vi "etc_XCITE_GetXCStruct.vi"(8 "error in (no error)":errorcluster {"code" format="%x"}, 11 "h":u64) -> (0 "error out":errorcluster {"code" format="%x"}, 1 "XCiteStructure":T1, 2 "ErrorMessage":i32 format="%x", 3 "h out":u64)   [LabVIEW 2019, in "XCite.lvlib"]
doc: "Gets the Xcite structure from the device with various properties."
uses:
  XCite.lvlib
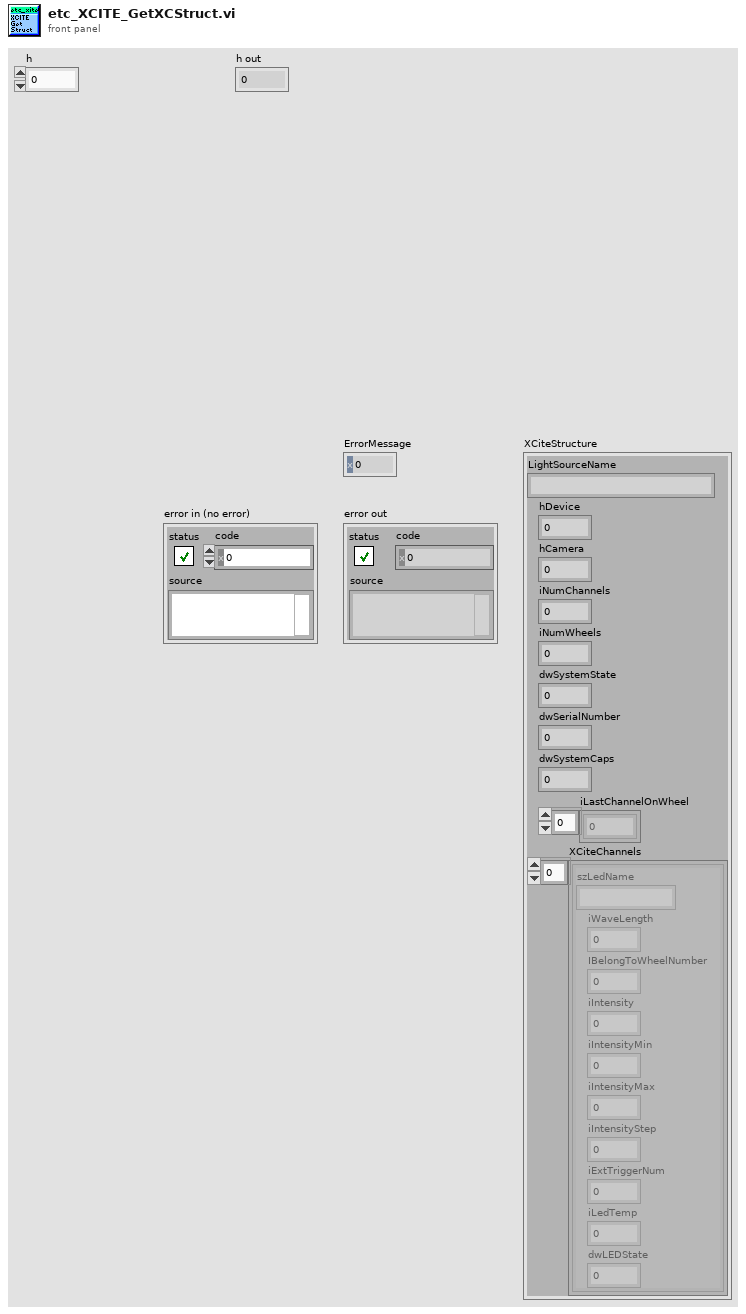
[diagram p1: front panel]
types:
  T1 = cluster{"LightSourceName":string, "hDevice":u64, "hCamera":u64, "iNumChannels":i32, "iNumWheels":i32, "dwSystemState":u32, "dwSerialNumber":u32, "dwSystemCaps":u32, "iLastChannelOnWheel":i16[], "XCiteChannels":cluster{"szLedName":string, "iWaveLength":i32, "IBelongToWheelNumber":i32, "iIntensity":i32, "iIntensityMin":i32, "iIntensityMax":i32, "iIntensityStep":i32, "iExtTriggerNum":i32, "iLedTemp":i32, "dwLEDState":u32}[]}
  T2 = cluster{"wSize":u16, "czLightSourceName":cluster{u8, u8, u8, u8, u8, u8, u8, u8, u8, u8, u8, u8, u8, u8, u8, u8, u8, u8, u8, u8, u8, u8, u8, u8, u8, u8, u8, u8, u8, u8}, "hDevice":u64, "hCamera":u64, "iNumChannels":i32, "iNumWheels":i32, "dwSystemState":u32, "dwSerialNumber":u32, "dwSystemCaps":u32, "iLastChannelOnWheel":cluster{i32, i32, i32, i32, i32}, "ZZdwDummy":cluster{u32, u32, u32, u32, u32, u32, u32, u32, u32, u32, u32, u32, u32, u32, u32, u32}, "XCiteChannels":cluster{"XCiteC_raw":cluster{"szLedName":cluster{u8, u8, u8, u8, u8, u8, u8, u8, u8, u8, u8, u8, u8, u8, u8, u8}, "iWaveLength":i32, "IBelongToWheelNumber":i32, "iIntensity":i32, "iIntensityMin":i32, "iIntensityMax":i32, "iIntensityStep":i32, "iExtTriggerNum":i32, "iLedTemp":i32, "dwLEDState":u32, "ZZdwdummy":cluster{u32, u32, u32, u32, u32, u32, u32, u32, u32, u32, u32, u32, u32, u32, u32, u32}}, "XCiteC_raw":cluster{"szLedName":cluster{u8, u8, u8, u8, u8, u8, u8, u8, u8, u8, u8, u8, u8, u8, u8, u8}, "iWaveLength":i32, "IBelongToWheelNumber":i32, "iIntensity":i32, "iIntensityMin":i32, "iIntensityMax":i32, "iIntensityStep":i32, "iExtTriggerNum":i32, "iLedTemp":i32, "dwLEDState":u32, "ZZdwdummy":cluster{u32, u32, u32, u32, u32, u32, u32, u32, u32, u32, u32, u32, u32, u32, u32, u32}}, "XCiteC_raw":cluster{"szLedName":cluster{u8, u8, u8, u8, u8, u8, u8, u8, u8, u8, u8, u8, u8, u8, u8, u8}, "iWaveLength":i32, "IBelongToWheelNumber":i32, "iIntensity":i32, "iIntensityMin":i32, "iIntensityMax":i32, "iIntensityStep":i32, "iExtTriggerNum":i32, "iLedTemp":i32, "dwLEDState":u32, "ZZdwdummy":cluster{u32, u32, u32, u32, u32, u32, u32, u32, u32, u32, u32, u32, u32, u32, u32, u32}}, "XCiteC_raw":cluster{"szLedName":cluster{u8, u8, u8, u8, u8, u8, u8, u8, u8, u8, u8, u8, u8, u8, u8, u8}, "iWaveLength":i32, "IBelongToWheelNumber":i32, "iIntensity":i32, "iIntensityMin":i32, "iIntensityMax":i32, "iIntensityStep":i32, "iExtTriggerNum":i32, "iLedTemp":i32, "dwLEDState":u32, "ZZdwdummy":cluster{u32, u32, u32, u32, u32, u32, u32, u32, u32, u32, u32, u32, u32, u32, u32, u32}}, "XCiteC_raw":cluster{"szLedName":cluster{u8, u8, u8, u8, u8, u8, u8, u8, u8, u8, u8, u8, u8, u8, u8, u8}, "iWaveLength":i32, "IBelongToWheelNumber":i32, "iIntensity":i32, "iIntensityMin":i32, "iIntensityMax":i32, "iIntensityStep":i32, "iExtTriggerNum":i32, "iLedTemp":i32, "dwLEDState":u32, "ZZdwdummy":cluster{u32, u32, u32, u32, u32, u32, u32, u32, u32, u32, u32, u32, u32, u32, u32, u32}}, "XCiteC_raw":cluster{"szLedName":cluster{u8, u8, u8, u8, u8, u8, u8, u8, u8, u8, u8, u8, u8, u8, u8, u8}, "iWaveLength":i32, "IBelongToWheelNumber":i32, "iIntensity":i32, "iIntensityMin":i32, "iIntensityMax":i32, "iIntensityStep":i32, "iExtTriggerNum":i32, "iLedTemp":i32, "dwLEDState":u32, "ZZdwdummy":cluster{u32, u32, u32, u32, u32, u32, u32, u32, u32, u32, u32, u32, u32, u32, u32, u32}}, "XCiteC_raw":cluster{"szLedName":cluster{u8, u8, u8, u8, u8, u8, u8, u8, u8, u8, u8, u8, u8, u8, u8, u8}, "iWaveLength":i32, "IBelongToWheelNumber":i32, "iIntensity":i32, "iIntensityMin":i32, "iIntensityMax":i32, "iIntensityStep":i32, "iExtTriggerNum":i32, "iLedTemp":i32, "dwLEDState":u32, "ZZdwdummy":cluster{u32, u32, u32, u32, u32, u32, u32, u32, u32, u32, u32, u32, u32, u32, u32, u32}}, "XCiteC_raw":cluster{"szLedName":cluster{u8, u8, u8, u8, u8, u8, u8, u8, u8, u8, u8, u8, u8, u8, u8, u8}, "iWaveLength":i32, "IBelongToWheelNumber":i32, "iIntensity":i32, "iIntensityMin":i32, "iIntensityMax":i32, "iIntensityStep":i32, "iExtTriggerNum":i32, "iLedTemp":i32, "dwLEDState":u32, "ZZdwdummy":cluster{u32, u32, u32, u32, u32, u32, u32, u32, u32, u32, u32, u32, u32, u32, u32, u32}}, "XCiteC_raw":cluster{"szLedName":cluster{u8, u8, u8, u8, u8, u8, u8, u8, u8, u8, u8, u8, u8, u8, u8, u8}, "iWaveLength":i32, "IBelongToWheelNumber":i32, "iIntensity":i32, "iIntensityMin":i32, "iIntensityMax":i32, "iIntensityStep":i32, "iExtTriggerNum":i32, "iLedTemp":i32, "dwLEDState":u32, "ZZdwdummy":cluster{u32, u32, u32, u32, u32, u32, u32, u32, u32, u32, u32, u32, u32, u32, u32, u32}}, "XCiteC_raw":cluster{"szLedName":cluster{u8, u8, u8, u8, u8, u8, u8, u8, u8, u8, u8, u8, u8, u8, u8, u8}, "iWaveLength":i32, "IBelongToWheelNumber":i32, "iIntensity":i32, "iIntensityMin":i32, "iIntensityMax":i32, "iIntensityStep":i32, "iExtTriggerNum":i32, "iLedTemp":i32, "dwLEDState":u32, "ZZdwdummy":cluster{u32, u32, u32, u32, u32, u32, u32, u32, u32, u32, u32, u32, u32, u32, u32, u32}}, "XCiteC_raw":cluster{"szLedName":cluster{u8, u8, u8, u8, u8, u8, u8, u8, u8, u8, u8, u8, u8, u8, u8, u8}, "iWaveLength":i32, "IBelongToWheelNumber":i32, "iIntensity":i32, "iIntensityMin":i32, "iIntensityMax":i32, "iIntensityStep":i32, "iExtTriggerNum":i32, "iLedTemp":i32, "dwLEDState":u32, "ZZdwdummy":cluster{u32, u32, u32, u32, u32, u32, u32, u32, u32, u32, u32, u32, u32, u32, u32, u32}}, "XCiteC_raw":cluster{"szLedName":cluster{u8, u8, u8, u8, u8, u8, u8, u8, u8, u8, u8, u8, u8, u8, u8, u8}, "iWaveLength":i32, "IBelongToWheelNumber":i32, "iIntensity":i32, "iIntensityMin":i32, "iIntensityMax":i32, "iIntensityStep":i32, "iExtTriggerNum":i32, "iLedTemp":i32, "dwLEDState":u32, "ZZdwdummy":cluster{u32, u32, u32, u32, u32, u32, u32, u32, u32, u32, u32, u32, u32, u32, u32, u32}}, "XCiteC_raw":cluster{"szLedName":cluster{u8, u8, u8, u8, u8, u8, u8, u8, u8, u8, u8, u8, u8, u8, u8, u8}, "iWaveLength":i32, "IBelongToWheelNumber":i32, "iIntensity":i32, "iIntensityMin":i32, "iIntensityMax":i32, "iIntensityStep":i32, "iExtTriggerNum":i32, "iLedTemp":i32, "dwLEDState":u32, "ZZdwdummy":cluster{u32, u32, u32, u32, u32, u32, u32, u32, u32, u32, u32, u32, u32, u32, u32, u32}}, "XCiteC_raw":cluster{"szLedName":cluster{u8, u8, u8, u8, u8, u8, u8, u8, u8, u8, u8, u8, u8, u8, u8, u8}, "iWaveLength":i32, "IBelongToWheelNumber":i32, "iIntensity":i32, "iIntensityMin":i32, "iIntensityMax":i32, "iIntensityStep":i32, "iExtTriggerNum":i32, "iLedTemp":i32, "dwLEDState":u32, "ZZdwdummy":cluster{u32, u32, u32, u32, u32, u32, u32, u32, u32, u32, u32, u32, u32, u32, u32, u32}}, "XCiteC_raw":cluster{"szLedName":cluster{u8, u8, u8, u8, u8, u8, u8, u8, u8, u8, u8, u8, u8, u8, u8, u8}, "iWaveLength":i32, "IBelongToWheelNumber":i32, "iIntensity":i32, "iIntensityMin":i32, "iIntensityMax":i32, "iIntensityStep":i32, "iExtTriggerNum":i32, "iLedTemp":i32, "dwLEDState":u32, "ZZdwdummy":cluster{u32, u32, u32, u32, u32, u32, u32, u32, u32, u32, u32, u32, u32, u32, u32, u32}}, "XCiteC_raw":cluster{"szLedName":cluster{u8, u8, u8, u8, u8, u8, u8, u8, u8, u8, u8, u8, u8, u8, u8, u8}, "iWaveLength":i32, "IBelongToWheelNumber":i32, "iIntensity":i32, "iIntensityMin":i32, "iIntensityMax":i32, "iIntensityStep":i32, "iExtTriggerNum":i32, "iLedTemp":i32, "dwLEDState":u32, "ZZdwdummy":cluster{u32, u32, u32, u32, u32, u32, u32, u32, u32, u32, u32, u32, u32, u32, u32, u32}}}}
  T3 = cluster{u8, u8, u8, u8, u8, u8, u8, u8, u8, u8, u8, u8, u8, u8, u8, u8, u8, u8, u8, u8, u8, u8, u8, u8, u8, u8, u8, u8, u8, u8}
  T4 = cluster{"XCiteC_raw":cluster{"szLedName":cluster{u8, u8, u8, u8, u8, u8, u8, u8, u8, u8, u8, u8, u8, u8, u8, u8}, "iWaveLength":i32, "IBelongToWheelNumber":i32, "iIntensity":i32, "iIntensityMin":i32, "iIntensityMax":i32, "iIntensityStep":i32, "iExtTriggerNum":i32, "iLedTemp":i32, "dwLEDState":u32, "ZZdwdummy":cluster{u32, u32, u32, u32, u32, u32, u32, u32, u32, u32, u32, u32, u32, u32, u32, u32}}, "XCiteC_raw":cluster{"szLedName":cluster{u8, u8, u8, u8, u8, u8, u8, u8, u8, u8, u8, u8, u8, u8, u8, u8}, "iWaveLength":i32, "IBelongToWheelNumber":i32, "iIntensity":i32, "iIntensityMin":i32, "iIntensityMax":i32, "iIntensityStep":i32, "iExtTriggerNum":i32, "iLedTemp":i32, "dwLEDState":u32, "ZZdwdummy":cluster{u32, u32, u32, u32, u32, u32, u32, u32, u32, u32, u32, u32, u32, u32, u32, u32}}, "XCiteC_raw":cluster{"szLedName":cluster{u8, u8, u8, u8, u8, u8, u8, u8, u8, u8, u8, u8, u8, u8, u8, u8}, "iWaveLength":i32, "IBelongToWheelNumber":i32, "iIntensity":i32, "iIntensityMin":i32, "iIntensityMax":i32, "iIntensityStep":i32, "iExtTriggerNum":i32, "iLedTemp":i32, "dwLEDState":u32, "ZZdwdummy":cluster{u32, u32, u32, u32, u32, u32, u32, u32, u32, u32, u32, u32, u32, u32, u32, u32}}, "XCiteC_raw":cluster{"szLedName":cluster{u8, u8, u8, u8, u8, u8, u8, u8, u8, u8, u8, u8, u8, u8, u8, u8}, "iWaveLength":i32, "IBelongToWheelNumber":i32, "iIntensity":i32, "iIntensityMin":i32, "iIntensityMax":i32, "iIntensityStep":i32, "iExtTriggerNum":i32, "iLedTemp":i32, "dwLEDState":u32, "ZZdwdummy":cluster{u32, u32, u32, u32, u32, u32, u32, u32, u32, u32, u32, u32, u32, u32, u32, u32}}, "XCiteC_raw":cluster{"szLedName":cluster{u8, u8, u8, u8, u8, u8, u8, u8, u8, u8, u8, u8, u8, u8, u8, u8}, "iWaveLength":i32, "IBelongToWheelNumber":i32, "iIntensity":i32, "iIntensityMin":i32, "iIntensityMax":i32, "iIntensityStep":i32, "iExtTriggerNum":i32, "iLedTemp":i32, "dwLEDState":u32, "ZZdwdummy":cluster{u32, u32, u32, u32, u32, u32, u32, u32, u32, u32, u32, u32, u32, u32, u32, u32}}, "XCiteC_raw":cluster{"szLedName":cluster{u8, u8, u8, u8, u8, u8, u8, u8, u8, u8, u8, u8, u8, u8, u8, u8}, "iWaveLength":i32, "IBelongToWheelNumber":i32, "iIntensity":i32, "iIntensityMin":i32, "iIntensityMax":i32, "iIntensityStep":i32, "iExtTriggerNum":i32, "iLedTemp":i32, "dwLEDState":u32, "ZZdwdummy":cluster{u32, u32, u32, u32, u32, u32, u32, u32, u32, u32, u32, u32, u32, u32, u32, u32}}, "XCiteC_raw":cluster{"szLedName":cluster{u8, u8, u8, u8, u8, u8, u8, u8, u8, u8, u8, u8, u8, u8, u8, u8}, "iWaveLength":i32, "IBelongToWheelNumber":i32, "iIntensity":i32, "iIntensityMin":i32, "iIntensityMax":i32, "iIntensityStep":i32, "iExtTriggerNum":i32, "iLedTemp":i32, "dwLEDState":u32, "ZZdwdummy":cluster{u32, u32, u32, u32, u32, u32, u32, u32, u32, u32, u32, u32, u32, u32, u32, u32}}, "XCiteC_raw":cluster{"szLedName":cluster{u8, u8, u8, u8, u8, u8, u8, u8, u8, u8, u8, u8, u8, u8, u8, u8}, "iWaveLength":i32, "IBelongToWheelNumber":i32, "iIntensity":i32, "iIntensityMin":i32, "iIntensityMax":i32, "iIntensityStep":i32, "iExtTriggerNum":i32, "iLedTemp":i32, "dwLEDState":u32, "ZZdwdummy":cluster{u32, u32, u32, u32, u32, u32, u32, u32, u32, u32, u32, u32, u32, u32, u32, u32}}, "XCiteC_raw":cluster{"szLedName":cluster{u8, u8, u8, u8, u8, u8, u8, u8, u8, u8, u8, u8, u8, u8, u8, u8}, "iWaveLength":i32, "IBelongToWheelNumber":i32, "iIntensity":i32, "iIntensityMin":i32, "iIntensityMax":i32, "iIntensityStep":i32, "iExtTriggerNum":i32, "iLedTemp":i32, "dwLEDState":u32, "ZZdwdummy":cluster{u32, u32, u32, u32, u32, u32, u32, u32, u32, u32, u32, u32, u32, u32, u32, u32}}, "XCiteC_raw":cluster{"szLedName":cluster{u8, u8, u8, u8, u8, u8, u8, u8, u8, u8, u8, u8, u8, u8, u8, u8}, "iWaveLength":i32, "IBelongToWheelNumber":i32, "iIntensity":i32, "iIntensityMin":i32, "iIntensityMax":i32, "iIntensityStep":i32, "iExtTriggerNum":i32, "iLedTemp":i32, "dwLEDState":u32, "ZZdwdummy":cluster{u32, u32, u32, u32, u32, u32, u32, u32, u32, u32, u32, u32, u32, u32, u32, u32}}, "XCiteC_raw":cluster{"szLedName":cluster{u8, u8, u8, u8, u8, u8, u8, u8, u8, u8, u8, u8, u8, u8, u8, u8}, "iWaveLength":i32, "IBelongToWheelNumber":i32, "iIntensity":i32, "iIntensityMin":i32, "iIntensityMax":i32, "iIntensityStep":i32, "iExtTriggerNum":i32, "iLedTemp":i32, "dwLEDState":u32, "ZZdwdummy":cluster{u32, u32, u32, u32, u32, u32, u32, u32, u32, u32, u32, u32, u32, u32, u32, u32}}, "XCiteC_raw":cluster{"szLedName":cluster{u8, u8, u8, u8, u8, u8, u8, u8, u8, u8, u8, u8, u8, u8, u8, u8}, "iWaveLength":i32, "IBelongToWheelNumber":i32, "iIntensity":i32, "iIntensityMin":i32, "iIntensityMax":i32, "iIntensityStep":i32, "iExtTriggerNum":i32, "iLedTemp":i32, "dwLEDState":u32, "ZZdwdummy":cluster{u32, u32, u32, u32, u32, u32, u32, u32, u32, u32, u32, u32, u32, u32, u32, u32}}, "XCiteC_raw":cluster{"szLedName":cluster{u8, u8, u8, u8, u8, u8, u8, u8, u8, u8, u8, u8, u8, u8, u8, u8}, "iWaveLength":i32, "IBelongToWheelNumber":i32, "iIntensity":i32, "iIntensityMin":i32, "iIntensityMax":i32, "iIntensityStep":i32, "iExtTriggerNum":i32, "iLedTemp":i32, "dwLEDState":u32, "ZZdwdummy":cluster{u32, u32, u32, u32, u32, u32, u32, u32, u32, u32, u32, u32, u32, u32, u32, u32}}, "XCiteC_raw":cluster{"szLedName":cluster{u8, u8, u8, u8, u8, u8, u8, u8, u8, u8, u8, u8, u8, u8, u8, u8}, "iWaveLength":i32, "IBelongToWheelNumber":i32, "iIntensity":i32, "iIntensityMin":i32, "iIntensityMax":i32, "iIntensityStep":i32, "iExtTriggerNum":i32, "iLedTemp":i32, "dwLEDState":u32, "ZZdwdummy":cluster{u32, u32, u32, u32, u32, u32, u32, u32, u32, u32, u32, u32, u32, u32, u32, u32}}, "XCiteC_raw":cluster{"szLedName":cluster{u8, u8, u8, u8, u8, u8, u8, u8, u8, u8, u8, u8, u8, u8, u8, u8}, "iWaveLength":i32, "IBelongToWheelNumber":i32, "iIntensity":i32, "iIntensityMin":i32, "iIntensityMax":i32, "iIntensityStep":i32, "iExtTriggerNum":i32, "iLedTemp":i32, "dwLEDState":u32, "ZZdwdummy":cluster{u32, u32, u32, u32, u32, u32, u32, u32, u32, u32, u32, u32, u32, u32, u32, u32}}, "XCiteC_raw":cluster{"szLedName":cluster{u8, u8, u8, u8, u8, u8, u8, u8, u8, u8, u8, u8, u8, u8, u8, u8}, "iWaveLength":i32, "IBelongToWheelNumber":i32, "iIntensity":i32, "iIntensityMin":i32, "iIntensityMax":i32, "iIntensityStep":i32, "iExtTriggerNum":i32, "iLedTemp":i32, "dwLEDState":u32, "ZZdwdummy":cluster{u32, u32, u32, u32, u32, u32, u32, u32, u32, u32, u32, u32, u32, u32, u32, u32}}}
  T5 = cluster{"szLedName":string, "iWaveLength":i32, "IBelongToWheelNumber":i32, "iIntensity":i32, "iIntensityMin":i32, "iIntensityMax":i32, "iIntensityStep":i32, "iExtTriggerNum":i32, "iLedTemp":i32, "dwLEDState":u32}[]
  T6 = cluster{"szLedName":cluster{u8, u8, u8, u8, u8, u8, u8, u8, u8, u8, u8, u8, u8, u8, u8, u8}, "iWaveLength":i32, "IBelongToWheelNumber":i32, "iIntensity":i32, "iIntensityMin":i32, "iIntensityMax":i32, "iIntensityStep":i32, "iExtTriggerNum":i32, "iLedTemp":i32, "dwLEDState":u32, "ZZdwdummy":cluster{u32, u32, u32, u32, u32, u32, u32, u32, u32, u32, u32, u32, u32, u32, u32, u32}}[]
  T7 = cluster{u8, u8, u8, u8, u8, u8, u8, u8, u8, u8, u8, u8, u8, u8, u8, u8}
  T8 = cluster{"szLedName":string, "iWaveLength":i32, "IBelongToWheelNumber":i32, "iIntensity":i32, "iIntensityMin":i32, "iIntensityMax":i32, "iIntensityStep":i32, "iExtTriggerNum":i32, "iLedTemp":i32, "dwLEDState":u32}
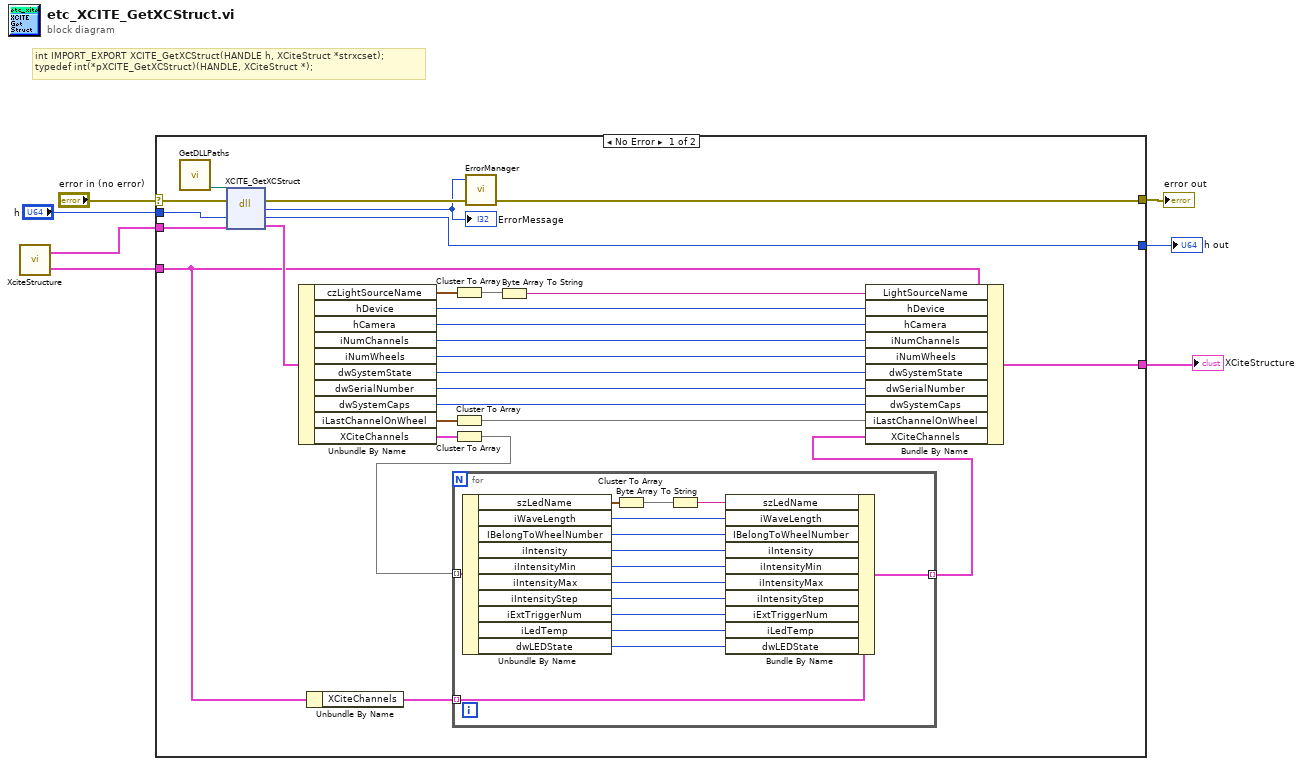
[diagram p0: block diagram]
diagram:
  # "int IMPORT_EXPORT XCITE_GetXCStruct(HANDLE h, XCiteStruct *strxcset);\ntypedef int(*pXCITE_GetXCStruct)(HANDLE, XCiteStruct *);"
  n1 = call "XciteStructure.vi"() -> ("XCiteStruct"=w3:T1, "XCiteStructure_raw"=w2:T2)  [unwired: 4 in, 2 out]
  n2 = case shown="No Error" "error in (no error)" {
    selector: "error in (no error)" -> [w34 w52]
    tunnel: [w32 w52] -> w7
    tunnel: "h" -> [w30 w51]
    tunnel: [w29 w51] -> w5
    tunnel: w2 -> [w27 _]
    tunnel: w3 -> [w12 w50]
    tunnel: [w8 w50] -> w1
    frame No Error {
      n3 = call "GetDLLPaths.vi"() -> ("etc_xcite_path"=w28:path)  [unwired: 8 in, 3 out]
      n4 = dll-call lib="C:/LabVIEWDevFall2024/pco.labview/labview_sdk/runtime/bin64/etc_xcite.dll" fn="XCITE_GetXCStruct"(path in=w28, error in=w34, "h"=w30, "XciteStucture"=w27) -> (error out=w33:errorcluster, "return type"=w31:i32, "h"=w29:u64, "XciteStucture"=w26:T2)  [unwired: 1 in, 1 out]
      "ErrorMessage" <- w31
      n5 = Unbundle By Name(w26) -> ("czLightSourceName"=w23:T3, "hDevice"=w19:u64, "hCamera"=w18:u64, "iNumChannels"=w17:i32, "iNumWheels"=w16:i32, "dwSystemState"=w15:u32, "dwSerialNumber"=w14:u32, "dwSystemCaps"=w13:u32, "iLastChannelOnWheel"=w25:cluster{i32, i32, i32, i32, i32}, "XCiteChannels"=w24:T4)
      n6 = Unbundle By Name(w12) -> ("XCiteChannels"=w11:T5)
      n7 = Cluster To Array(cluster=w23) -> (array=w22:u8[])
      n8 = Cluster To Array(cluster=w25) -> (array=w20:i32[])
      n9 = Cluster To Array(cluster=w24) -> (array=w10:T6)
      n10 = for {
        tunnel: w11 -> [w48] mode=indexing
        tunnel: w10 -> [w49] mode=indexing
        tunnel: [w35] -> w9 mode=indexing
        n11 = Unbundle By Name(w49) -> ("szLedName"=w47:T7, "iWaveLength"=w44:i32, "IBelongToWheelNumber"=w43:i32, "iIntensity"=w42:i32, "iIntensityMin"=w41:i32, "iIntensityMax"=w40:i32, "iIntensityStep"=w39:i32, "iExtTriggerNum"=w38:i32, "iLedTemp"=w37:i32, "dwLEDState"=w36:u32)
        n12 = Cluster To Array(cluster=w47) -> (array=w46:u8[])
        n13 = Byte Array To String(unsigned byte array=w46) -> (string=w45:string)
        n14 = Bundle By Name(cluster=w48, "szLedName"=w45, "iWaveLength"=w44, "IBelongToWheelNumber"=w43, "iIntensity"=w42, "iIntensityMin"=w41, "iIntensityMax"=w40, "iIntensityStep"=w39, "iExtTriggerNum"=w38, "iLedTemp"=w37, "dwLEDState"=w36) -> (w35:T8)
      }
      n15 = call "ErrorManager.vi"("error in (no error)"=w33, "error code"=w31) -> ("error out"=w32:errorcluster)  [unwired: 2 in, 1 out]
      n16 = Byte Array To String(unsigned byte array=w22) -> (string=w21:string)
      n17 = Bundle By Name(cluster=w12, "LightSourceName"=w21, "hDevice"=w19, "hCamera"=w18, "iNumChannels"=w17, "iNumWheels"=w16, "dwSystemState"=w15, "dwSerialNumber"=w14, "dwSystemCaps"=w13, "iLastChannelOnWheel"=w20, "XCiteChannels"=w9) -> (w8:T1)
    }
    frame Error {
    }
  }
  "error out" <- w7
  "h out" <- w5
  "XCiteStructure" <- w1
